vi "Save File Globals HCC.vi"() -> ()   [LabVIEW 2023]
panel:
  out "Heating":u32(colorbox)=15688704
  out "Problem":u32(colorbox)=15012864
  out "Pause":u32(colorbox)=14927872
  out "Run":u32(colorbox)=6334743
  out "EOC":u32(colorbox)=20719
  in  "Color Uncofigured":u32(colorbox)=7171459
  in  "Startup":u32(colorbox)
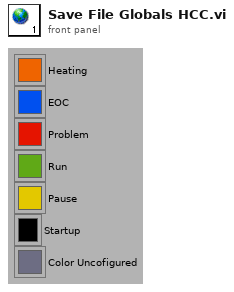
[diagram p1: front panel]
diagram:
